vi "Worked Example--Pressure Units Converter.vi"() -> ()   [LabVIEW 2013]
panel:
  in  "Output Units":T1(radio)=enum."Pascals (Pa)"
  in  "Input Units":T1(radio)=enum."inches of mercury (inHg)"
  out "Converted Value:":dbl=101325.0
  in  "Input Value:":dbl=29.92126
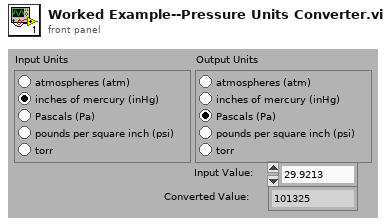
[diagram p1: front panel]
types:
  T1 = enum32{"atmospheres (atm)", "inches of mercury (inHg)", "Pascals (Pa)", "pounds per square inch (psi)", "torr"}
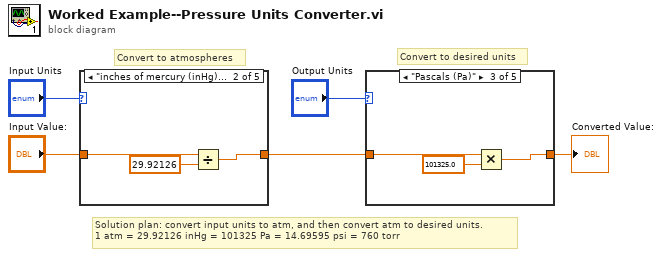
[diagram p0: block diagram]
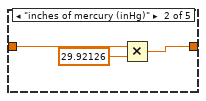
[diagram p3: hidden frame]
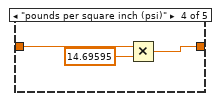
[diagram p4: hidden frame]
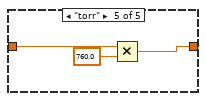
[diagram p5: hidden frame]
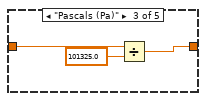
[diagram p7: hidden frame]
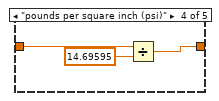
[diagram p8: hidden frame]
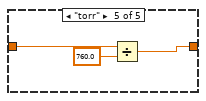
[diagram p9: hidden frame]
diagram:
  # "Convert to desired units"
  # "Convert to atmospheres"
  # "Solution plan: convert input units to atm, and then convert atm to desired units.\n1 atm = 29.92126 inHg = 101325 Pa = 14.69595 psi = 760 torr"
  n1 = case shown="\"inches of mercury (inHg)\"" "Input Units" {
    tunnel: "Input Value:" -> [w6 w9 w11 w14 w17]
    tunnel: [w6 w8 w10 w13 w16] -> w2
    frame "atmospheres (atm)", Default {
    }
    frame "inches of mercury (inHg)" {
      n2 = Divide(x=w9, y=29.92126) -> (x/y=w8:dbl)
    }
    frame "Pascals (Pa)" {
      n3 = Divide(x=w11, y=101325.0) -> (x/y=w10:dbl)
    }
    frame "pounds per square inch (psi)" {
      n4 = Divide(x=w14, y=14.69595) -> (x/y=w13:dbl)
    }
    frame "torr" {
      n5 = Divide(x=w17, y=760.0) -> (x/y=w16:dbl)
    }
  }
  n6 = case shown="\"Pascals (Pa)\"" "Output Units" {
    tunnel: w2 -> [w19 w22 w24 w27 w30]
    tunnel: [w19 w21 w23 w26 w29] -> w1
    frame "atmospheres (atm)", Default {
    }
    frame "inches of mercury (inHg)" {
      n7 = Multiply(x=w22, y=29.92126) -> (x*y=w21:dbl)
    }
    frame "Pascals (Pa)" {
      n8 = Multiply(x=w24, y=101325.0) -> (x*y=w23:dbl)
    }
    frame "pounds per square inch (psi)" {
      n9 = Multiply(x=w27, y=14.69595) -> (x*y=w26:dbl)
    }
    frame "torr" {
      n10 = Multiply(x=w30, y=760.0) -> (x*y=w29:dbl)
    }
  }
  "Converted Value:" <- w1
